vi "Init.vi"(8 "error in (no error)":errorcluster, 10 "Group Config":refnum<class "Group Config.lvclass">) -> (0 "error out":errorcluster, 3 "Group":refnum<class "Group.lvclass">)   [LabVIEW 2020, in "Vecto.lvlib" / "Group.lvclass"]
uses:
  Group.lvclass
  Group Config/Group Config.lvclass
  Group Config/Group Config.lvclass/Group Config.ctl
  Group DBL/Group DBL.lvclass
  C:/dev/lv20CE/relink/lv-vecto/Vecto/Group/Group.lvclass
  Group STR/Group STR.lvclass
  Group BOOL/Group BOOL.lvclass
  Ref.ctl
  Channel Info.ctl
  Group.lvclass/Group.ctl
  01584b93-a09b-41fa-a727-74251d7e872a.vi
  VectoConfig/VectoConfig.lvlib
  Channel Config/Channel Config.lvclass
  Vecto.lvlib
  C:/dev/lv20CE/relink/lv-vecto/Vecto/Group DBL/Group DBL.lvclass
  C:/dev/lv20CE/relink/lv-vecto/Vecto/Group STR/Group STR.lvclass
  C:/dev/lv20CE/relink/lv-vecto/Vecto/Group BOOL/Group BOOL.lvclass
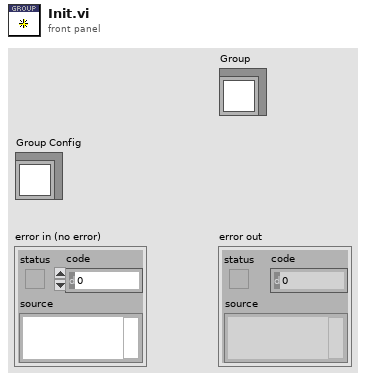
[diagram p1: front panel]
types:
  T1 = typedef "VectoConfig.lvlib/Channel Info.ctl" = cluster{"Name":string, "Group":string, "Owning Node":string, "Owning Task":string, "Resource":string}
  T2 = typedef "VectoConfig.lvlib/Group Data Type.ctl" = enum16{"Double", "String", "Bool"}
  T3 = typedef "Vecto.lvlib/Group.lvclass/Ref.ctl" = cluster{"Channel Index Map":map{string, i32}, "Channel Info":T1[], "Bad":bool}
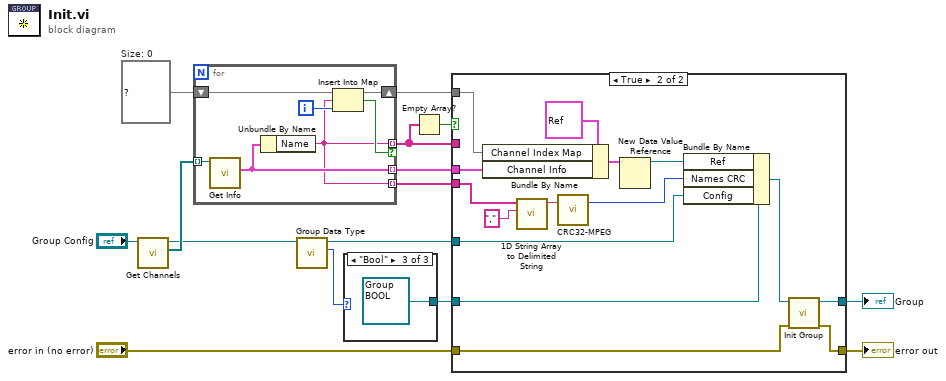
[diagram p0: block diagram]
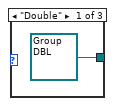
[diagram p2: hidden frame]
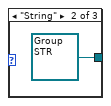
[diagram p3: hidden frame]
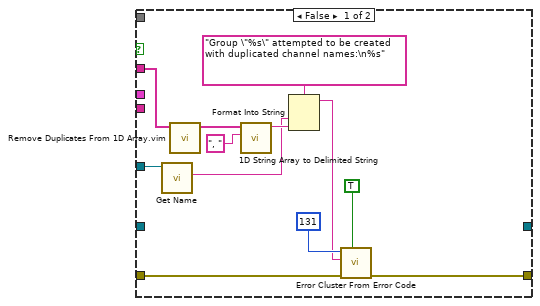
[diagram p4: hidden frame]
diagram:
  w15 = map{string, i32} {}  # Size: 0
  n1 = call "Get Channels.vi"("Group Config in"="Group Config") -> ("Channels"=w10:refnum<class "Channel Config.lvclass">[], "Group Config out"=w5:refnum<class "Group Config.lvclass">)  [unwired: 8 in, 1 out]
  n2 = for {
    tunnel: w10 -> [w18] mode=indexing
    tunnel: [w17] -> w13 mode=indexing
    shift-right: [w21] -> w14
    shift-left: w15 -> [w22]
    tunnel: [w16] -> w12 mode=indexing if=w20
    tunnel: [w16] -> w1 mode=indexing
    i -> [w19]
    n3 = call "Get Info.vi"("Channel Config in"=w18) -> ("Info"=w17:T1)  [unwired: 8 in, 2 out]
    n4 = Unbundle By Name(w17) -> ("Name"=w16:string)
    n5 = Insert Into Map(map in=w22, key=w16, value=w19) -> (map out=w21:map{string, i32}, key already included?=w20:bool)  [unwired: 1 out]
  }
  n6 = call "Group Data Type.vi"("Group Config in"=w5) -> ("Data Type"=w3:T2, "Group Config out"=w4:refnum<class "Group Config.lvclass">)  [unwired: 8 in, 1 out]
  n7 = case shown="\"Bool\"" w3 {
    tunnel: [refnum<class "Group DBL.lvclass"> refnum ("Vecto.lvlib:Group.lvclass") refnum<class "Group STR.lvclass"> refnum ("Vecto.lvlib:StringGroup.lvclass") refnum<class "Group BOOL.lvclass"> refnum ("Vecto.lvlib:Group BOOL.lvclass")] -> w2
    frame "Double" {
    }
    frame "String" {
    }
    frame "Bool" {
    }
  }
  n8 = Empty Array?(array=w12) -> (empty?=w11:bool)
  n9 = case shown="True" w11 {
    tunnel: [_ w48] -> w6
    tunnel: w4 -> [w27 w42]
    tunnel: "error in (no error)" -> [w37 w46]
    tunnel: [w30 w47] -> w7
    tunnel: w14 -> [_ w49]
    tunnel: w13 -> [_ w50]
    tunnel: w12 -> [w29 _]
    tunnel: w2 -> [_ w43]
    tunnel: w1 -> [_ w41]
    frame False {
      n10 = call "Get Name.vi"("Group Config in"=w27) -> ("Name"=w26:string)  [unwired: 8 in, 2 out]
      n11 = call "Remove Duplicates From 1D Array.vim"("array"=w29) -> ("array with duplicates removed"=w28:string[])  [unwired: 10 in]
      n12 = call <vilib>:"1D String Array to Delimited String.vi"("delimiter"=", ", "string array"=w28) -> ("delimited string"=w32:string)  [unwired: 9 in]
      n13 = Format Into String(format string="Group \"%s\" attempted to be created with duplicated channel names:\n%s", w26, w32) -> (resulting string=w31:string)  [unwired: 2 in, 1 out]
      n14 = call <vilib>:"Error Cluster From Error Code.vi"("show call chain? (False)"=TRUE, "error in (no error)"=w37, "error message (\"\")"=w31, "error code (0)"=131) -> ("error out"=w30:errorcluster)  [unwired: 5 in]
    }
    frame True {
      n15 = Bundle By Name(cluster=T3 {"Channel Index Map"={}, "Channel Info"=[], "Bad"=FALSE} ("Ref"), "Channel Index Map"=w49, "Channel Info"=w50) -> (w51:T3)
      n16 = call <vilib>:"1D String Array to Delimited String.vi"("delimiter"=",", "string array"=w41) -> ("delimited string"=w39:string)  [unwired: 9 in]
      n17 = call "CRC32-MPEG.vi"("Data In"=w39) -> ("CRC"=w38:u32)  [unwired: 6 in]
      n18 = New Data Value Reference(data value=w51) -> (data value reference=w44:refnum<data-value>)  [unwired: 1 in, 1 out]
      n19 = Bundle By Name(cluster=w43, "Ref"=w44, "Names CRC"=w38, "Config"=w42) -> (w45:refnum<class "Group.lvclass">)
      n20 = call-dynamic "Init Group.vi"("error in (no error)"=w46, "Group in"=w45) -> ("error out"=w47:errorcluster, "Group out"=w48:refnum<class "Group.lvclass">)  [unwired: 8 in]
    }
  }
  "error out" <- w7
  "Group" <- w6
